vi "1D String Array_DeleteEmptyCells.vi"(2 "1D String Array.IN":string[](array[string])=["30", ""]) -> (6 "1D String Array.OUT":string[](array[string])=["30", ""])   [LabVIEW 2020]
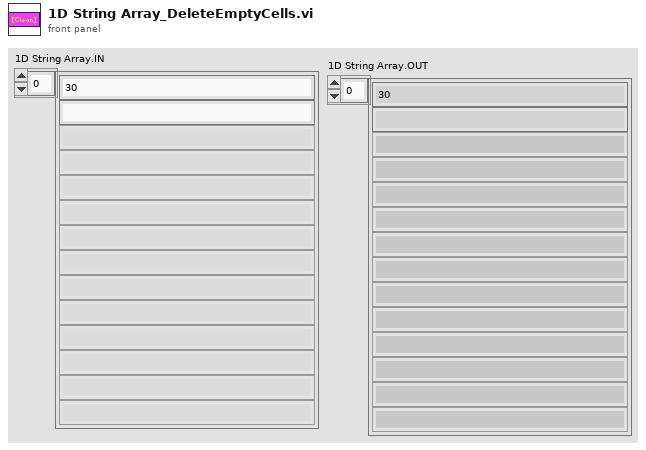
[diagram p1: front panel]
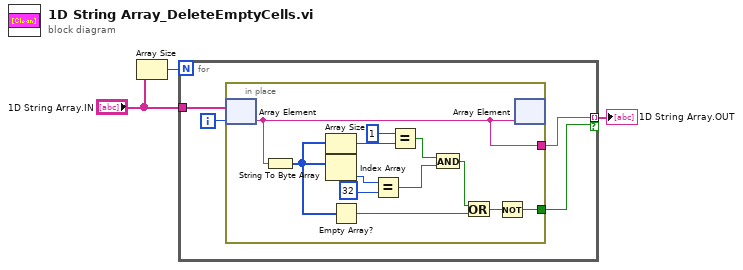
[diagram p0: block diagram]
diagram:
  n1 = Array Size(array="1D String Array.IN") -> (size(s)=w3:i32)
  n2 = for {
    N: w3 -> [_]
    tunnel: "1D String Array.IN" -> [w6]
    tunnel: [w4] -> w1 mode=indexing if=w7
    i -> [w5]
    n3 = in-place {
      in-place-border: [w9] -> w7
      in-place-border: [w8] -> w4
      n4 = in-place-array #1(w6, w5) -> (w8:string)
      n5 = String To Byte Array(string=w8) -> (unsigned byte array=w17:u8[])
      n6 = Array Size(array=w17) -> (size(s)=w16:i32)
      n7 = Index Array(array=w17) -> (element=w19:u8)  [unwired: 1 in]
      n8 = Empty Array?(array=w17) -> (empty?=w11:bool)
      n9 = Equal?(x=w19, y=u8 32) -> (x = y?=w13:bool)
      n10 = Equal?(x=1, y=w16) -> (x = y?=w14:bool)
      n11 = And(x=w14, y=w13) -> (x .and. y?=w12:bool)
      n12 = Or(x=w12, y=w11) -> (x .or. y?=w10:bool)
      n13 = Not(x=w10) -> (.not. x?=w9:bool)
      n14 = in-place-array #1(w8) -> ()  [unwired: 2 out]
    }
  }
  "1D String Array.OUT" <- w1
